vi "Dashboard 2022.vi"() -> ()   [LabVIEW 2020]
uses:
  <vilib>/event_ctls.llb/eventvkey.ctl
  <vilib>/Rock Robotics/WPI/Dashboard/WPI_DashboardLogging Global.vi
  <vilib>/Utility/miscctls.llb/LVRowAndColumnTypeDef.ctl
  <vilib>/Rock Robotics/Network Tables/NT Read Numeric Array.vi
panel:
  in  "Camera Settings Right":T1={"Frame Rate"=30, "Compression"=30, "Size"=1, "DB Camera Config"=FALSE} {"Frame Rate" scale=1.0..30.0; "Compression" scale=100.0..-1.0; "Size" items=["640x480", "320x240", "160x120"]}
  in  "Camera Name Right":string(combo)="No Camera Selection"
  out "Camera Perf":string
  in  "Camera Settings":T1={"Frame Rate"=30, "Compression"=30, "Size"=1, "DB Camera Config"=FALSE} {"Frame Rate" scale=1.0..30.0; "Compression" scale=100.0..-1.0; "Size" items=["640x480", "320x240", "160x120"]}
  in  "TCP":refnum<k5>
  in  "Rec Mode":enum32{"Stop", "Record", "Playback"}(radio)
  out "Robot IP":string
  out "Image Message":string="Timeout in Camera Communications"
  in  "Dashboard Tab":T2(tab)
  in  "Select Auto":string(combo)="Select Autonomous ..."
  out "NT Connection":bool
  out "MotorChart R":cluster{"Numeric":dbl, "Numeric":dbl}(graph)
  out "MotorChart L":cluster{"Numeric":dbl, "Numeric":dbl}(graph)
  out "MotorSliders R":cluster{"MotorSlide1":dbl, "MotorSlide2":dbl} {"MotorSlide2" scale=-1.0..1.0 scale format="%#_2e"; "MotorSlide1" scale=-1.0..1.0 scale format="%#_2e"}
  out "MotorSliders L":cluster{"MotorSlide1":dbl, "MotorSlide2":dbl} {"MotorSlide2" scale=-1.0..1.0 scale format="%#_2e"; "MotorSlide1" scale=-1.0..1.0 scale format="%#_2e"}
  out "Gyro":dbl(knob) scale=0.0..360.0
  out "JS1 Z":dbl(slide) scale=-1.0..1.0 scale format="%#_2e"
  out "JS1 Graph":cluster{"X":dbl, "Y":dbl}[](graph)
  out "JS1 Buttons":T3
  out "JS2 Z":dbl(slide) scale=-1.0..1.0 scale format="%#_2e"
  out "JS2 Graph":cluster{"X":dbl, "Y":dbl}[](graph)
  out "JS2 Buttons":T3
  out "Mode":T4(ring)=enum."Auto Disabled"
  out "Right Camera Perf":cluster{"Bandwidth (Mbps)":dbl, "FPS":dbl}
  out "Camera Image Right":T5(plugin-control)
  in  "DB/String 9":string
  in  "DB/String 8":string
  in  "DB/String 7":string
  in  "DB/String 6":string
  in  "DB/String 5":string
  in  "DB/String 4":string
  in  "DB/String 3":string
  in  "DB/String 2":string
  in  "DB/String 1":string
  in  "DB/String 0":string
  in  "DB/Slider 0":dbl(slide) scale=0.0..5.0
  in  "DB/Slider 1":dbl(slide) scale=0.0..5.0
  in  "DB/Slider 2":dbl(slide) scale=0.0..5.0
  in  "DB/Slider 3":dbl(slide) scale=0.0..5.0
  out "DB/LED 3":bool
  out "DB/LED 2":bool
  out "DB/LED 1":bool
  out "DB/LED 0":bool
  in  "DB/Button 3":bool
  in  "DB/Button 2":bool
  in  "DB/Button 1":bool
  in  "DB/Button 0":bool caption="New Name"
  in  "Test Slider":dbl(slide) scale=0.0..100.0 scale format="%#_3g"
  in  "On/Off":bool caption="Solenoid"
  in  "Test Name":u16(ring) items=["Select the test to run..."]
  in  "Test Tree":string(tree)
  in  "Motor":cluster{"Value":dbl, "Enable":bool} {"Value" scale=-1.0..1.0 scale format="%#_3g"}
  out "Progress":T6 {"Test Progress" scale=0.0..100.0}
  in  "Rev/Fwd":cluster{"Forward":bool, "Reverse":bool}
  in  "Test Ring":u16(ring) items=["Monochrome", "Color"]
  out "Cmd Status":string
  in  "Execute Command":bool
  in  "Command Params":string[][](table)
  in  "Command Selection":i32(listbox)
  in  "CheckList":i32(listbox)
  out "Tree":string(tree)
  out "Right Speed Chart":dbl(graph)
  out "Left Speed Chart":dbl(graph)
  out "Camera Image":T5(plugin-control)
  out "Background":bool
  in  "Camera Name":string(combo)="No Camera Selection"
  # "HW"
  # "HW"
  # "Joysticks"
  # "Drive Motors"
  # "Front"
  # "Right"
  # "Left"
  # "Back"
  # "This tab is a great place for autonomous settings and robot-specific values.\nPlace controls and indicators inside this tab and match name to\nDashboard Variables on robot. You can also delete this comment."
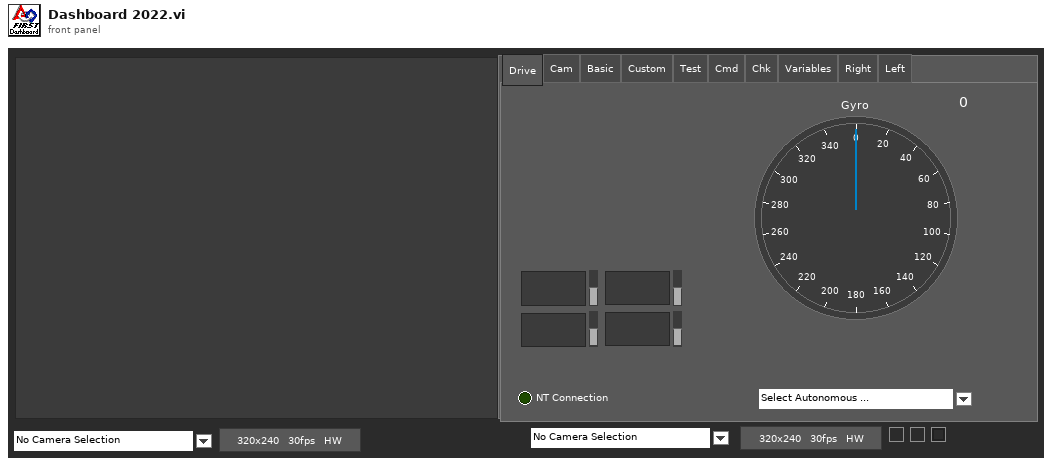
[diagram p1: front panel]
types:
  T1 = cluster{"Frame Rate":i32, "Compression":i32, "Size":u16, "DB Camera Config":bool}
  T2 = enum32{"Drive", "Cam", "Basic", "Custom", "Test", "Cmd", "Chk", "Variables", "Right", "Left"}
  T3 = cluster{bool, bool, bool, bool, bool, bool, bool, bool, bool, bool, bool, bool}
  T4 = enum8{"Tele-Op Disabled", "Tele-Op Enabled", "Auto Disabled", "Auto Enabled", "Test Disabled", "Test Enabled", "Disconnected", "No Code", "E-Stop"}
  T5 = typedef "IMAQ Image.ctl" = refnum<image>
  T6 = cluster{"Test Progress":u8, "Test Progress Text":string}
  T7 = cluster{"Save Path":path, "Interval (s)":dbl, "Keep":i32}
  T8 = enum32{"Drive", "Camera", "Basic", "Custom", "Test", "Commands", "Checklist", "Variables"}
  T9 = typedef "Image Type" = u32
  T10 = cluster{"IDs":cluster{"RPC field ID":u16, "Unique ID":u16}, "String":string}
  T11 = cluster{"Error Strings":string, "Disable Counts":cluster{u16, u16}, "Rail Faults":cluster{u16, u16, u16}, "Robot IP":string, "DB Mode":u8, "Event Info":cluster{"Name":string, "Type":u8, "Number":u16, "Replay":u8}}
  T12 = cluster{"Storage":cluster{"Disk Free":u64, "RAM Block":u32, "RAM free":u32}, "CPU Utilization":cluster{"CPU % ISR":sgl, "CPU % Time Crit":sgl, "CPU % Timed Str":sgl, "CPU % High":sgl, "CPU % Above":sgl, "CPU % Normal":sgl, "CPU % Low":sgl}, "CAN":cluster{"% Bus Utilization":sgl, "Bus Off Cnt":u32, "TX_FIFO Full Cnt":u32, "Receive Error Cnt":u8, "Transmit Error Cnt":u8}, "HID":cluster{"HID Outputs":u32, "Rumble Low":u16, "Rumble High":u16}[]}
  T13 = cluster{"Status bits":cluster{"Test Mode":bool, "Autonomous":bool, "Enabled":bool, "Code Start":bool, "Brownout":bool, "Reserved 2":bool, "Reserved 3":bool, "E-Stop":bool}, "Code Trace":cluster{"Disabled":bool, "TeleOp":bool, "Auto":bool, "Test":bool}, "Controller Type":enum16{"unknown", "cRIO", "roboRio"}, "Code?":enum16{"unknown", "noCode", "code"}, "Battery V":dbl}
  T14 = cluster{"Control Bits":cluster{"TestMode":bool, "Autonomous":bool, "Enabled":bool, "FMS Present":bool, bool, bool, bool, "E-Stop":bool}, "Team Station ":u8, "Countdown":sgl, "Joystick Values":cluster{"Axes":dbl[], "Buttons":bool[], "POVs":i16[]}[]}
  T15 = cluster{"Axes":dbl[], "Buttons":bool[], "POVs":i16[]}[]
  T16 = cluster{"Axes":dbl[], "Buttons":bool[], "POVs":i16[]}
  T17 = cluster{"Buttons[0]":bool, "Buttons[1]":bool, "Buttons[2]":bool, "Buttons[3]":bool, "Buttons[4]":bool, "Buttons[5]":bool, "Buttons[6]":bool, "Buttons[7]":bool, "Buttons[8]":bool, "Buttons[9]":bool, "Buttons[10]":bool, "Buttons[11]":bool}
  T18 = cluster{"Camera Image":refnum<vi>, "Dashboard Tab":refnum<vi>, "Background":refnum<vi>, "Rec Mode":refnum<vi>, "Test Slider":refnum<vi>, "On/Off ":refnum<vi>, "Test Ring":refnum<vi>, "Rev/Fwd":refnum<vi>, "Test Name":refnum<vi>, "Motor":refnum<vi>, "Progress":refnum<vi>, "CheckList":refnum<vi>, "Tree":refnum<vi>, "Test Tree":refnum<vi>, "Command Params":refnum<vi>, "Command Selection":refnum<vi>, "Execute Command":refnum<vi>, "Cmd Status":refnum<vi>, "Camera Settings":refnum<vi>, "Camera Name":refnum<vi>, "Camera Perf":refnum<vi>, "Camera Settings Right":refnum<vi>, "Camera Name Right":refnum<vi>, "Camera Image Right":refnum<vi>}
  T19 = cluster{"Global Rectangle":i32[], "Contours":cluster{"Contour Type":u32, "ROI Type":u32, "Points":i32[]}[]}
  T20 = cluster{"Camera Name":string, string, "Saved DB Images Info":cluster{"Save Path":path, "Interval (s)":dbl, "Keep":i32}}
  T21 = cluster{"Camera Name Right":string, string, "Saved DB Images Info":cluster{"Save Path":path, "Interval (s)":dbl, "Keep":i32}}
  T22 = cluster{"Operation":enum16{"Update", "Clear"}, "Color Box":u32}[]
  T23 = typedef "eventvkey.ctl" = enum16{"ASCII", "Enter", "Return", "Shift", "Ctrl", "Alt", "Cmd", "Opt", "Caps", "NumLock", "Clear", "Break", "Up", "Down", "Left", "Right", "Insert", "Delete", "Home", "End", "PageUp", "PageDown", "Escape", "Help", "Pause", "ScrollLock", "F1", "F2", "F3", "F4", "F5", "F6", "F7", "F8", "F9", "F10", "F11", "F12", "F13", "F14", "F15", "F16", "F17", "F18", "F19", "F20", "F21", "F22", "F23", "F24", "Play", "VolumeUp", "VolumeDown", "Mute", "Two Byte Char"}
  T24 = cluster{"Image Size":bool, "Image Type":bool, "Pixel Value":bool, "ROI Information":bool, "Zoom Factor":bool}
  T25 = cluster{"Operation":enum16{"Update", "Clear"}, "Color Box":u32}
  T26 = typedef "LVRowAndColumnTypeDef.ctl" = cluster{"Row":i32, "Column":i32}
  T27 = cluster{"Shift":bool, "Ctrl":bool, "Alt":bool, "Cmd":bool, "Opt":bool}
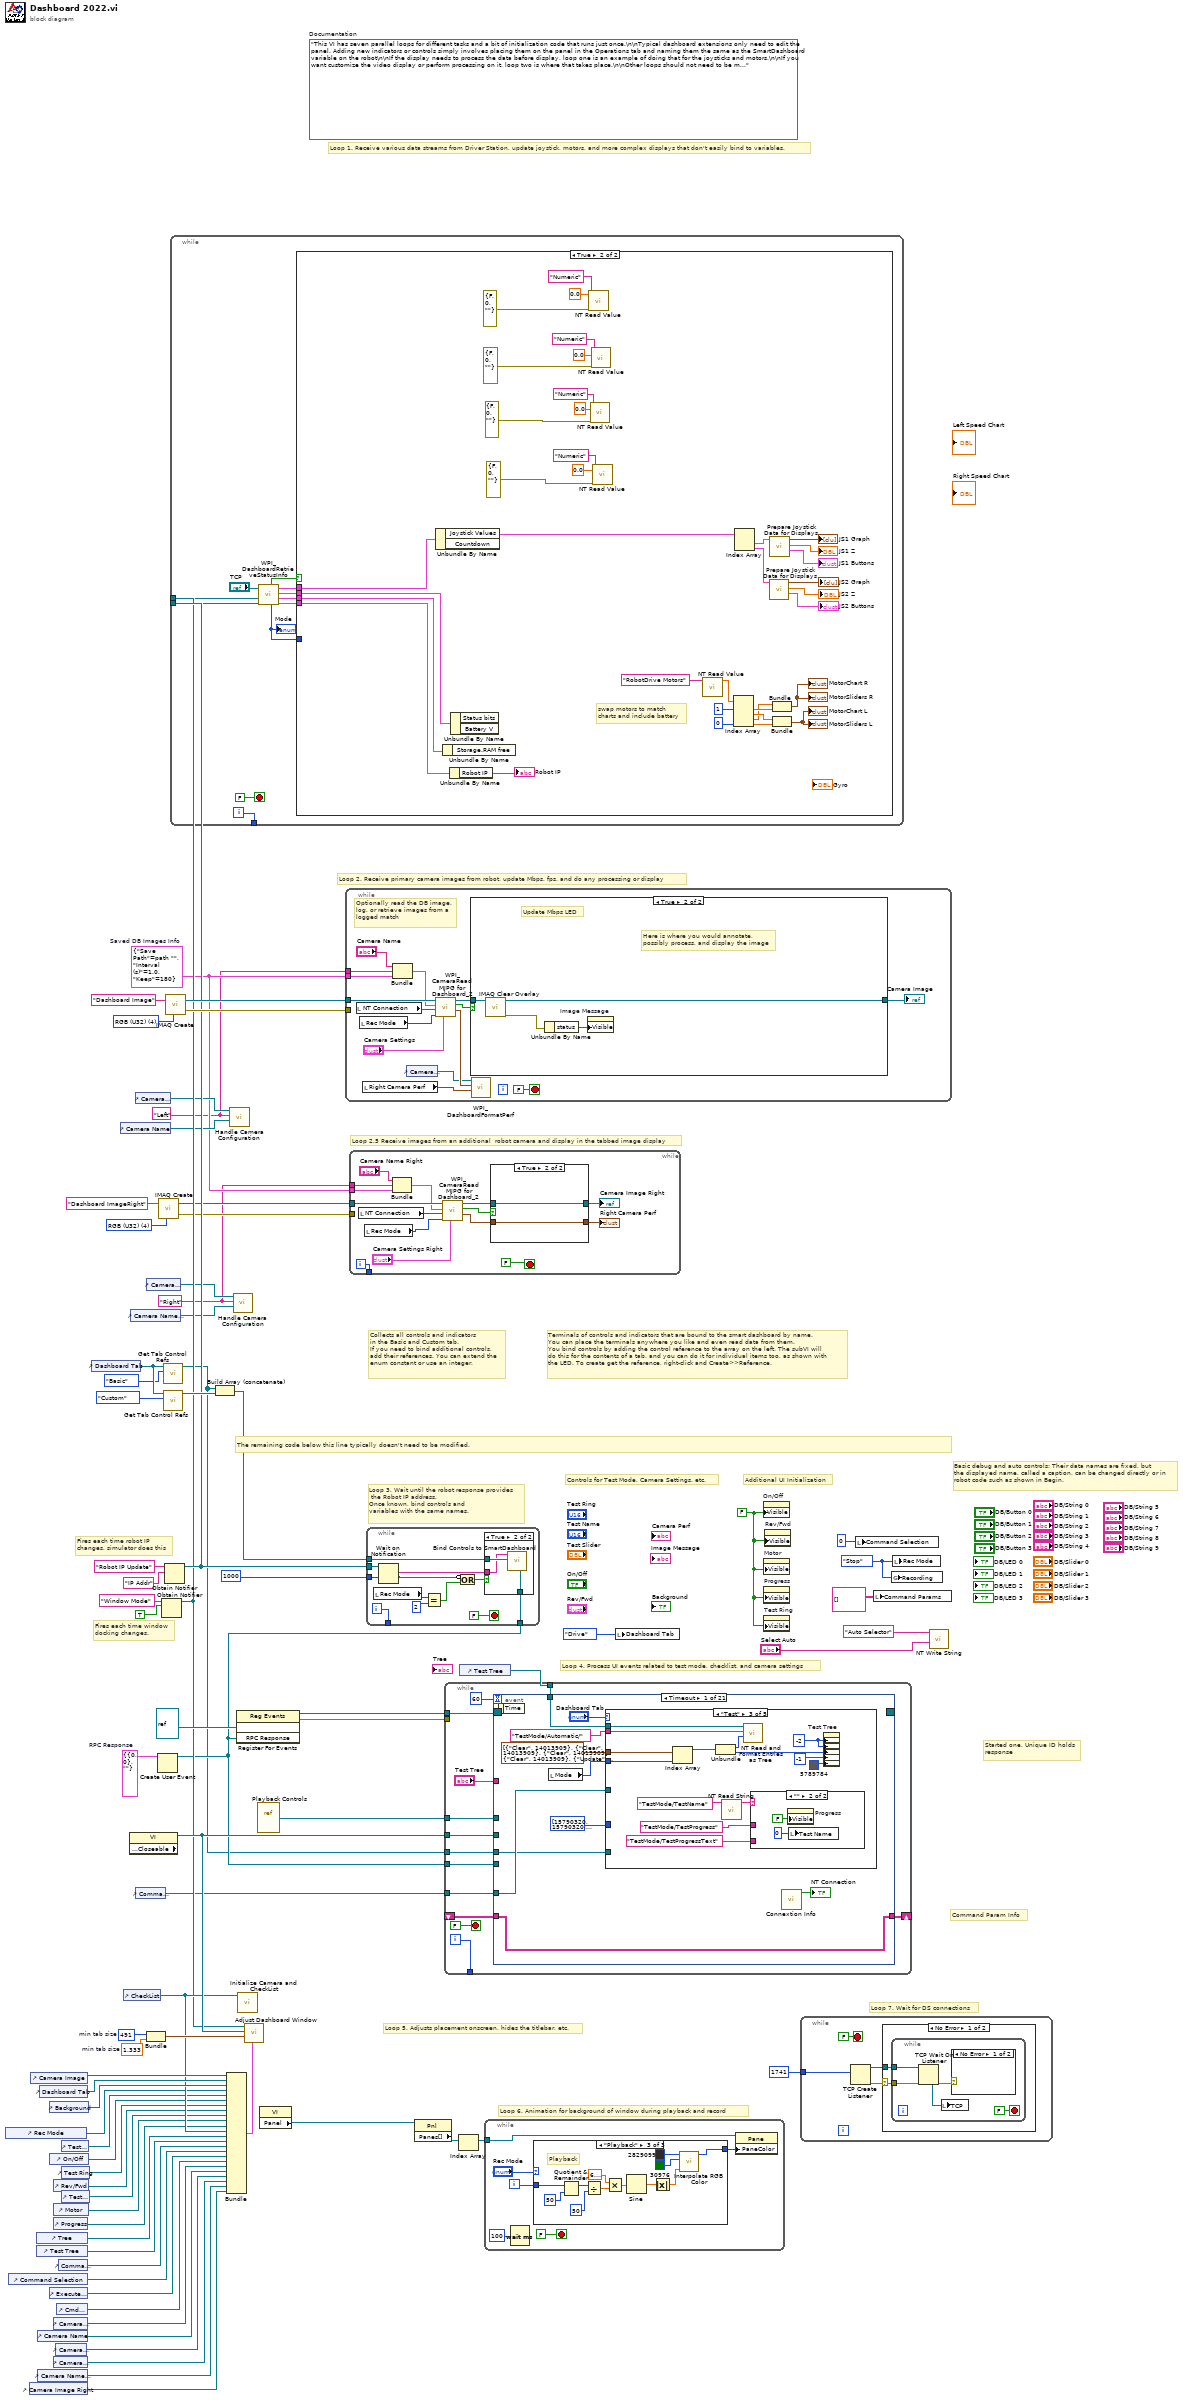
[diagram p0: block diagram]
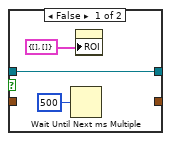
[diagram p2: hidden frame]
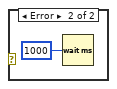
[diagram p3: hidden frame]
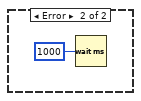
[diagram p4: hidden frame]
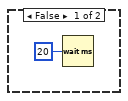
[diagram p5: hidden frame]
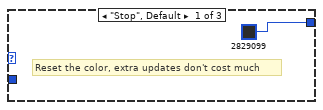
[diagram p6: hidden frame]
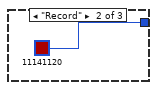
[diagram p7: hidden frame]
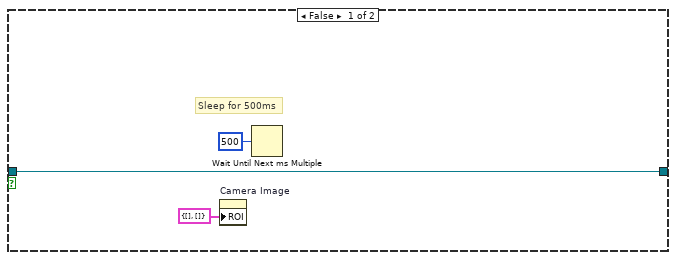
[diagram p9: hidden frame]
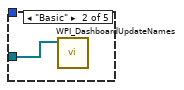
[diagram p11: hidden frame]
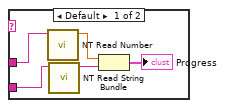
[diagram p12: hidden frame]
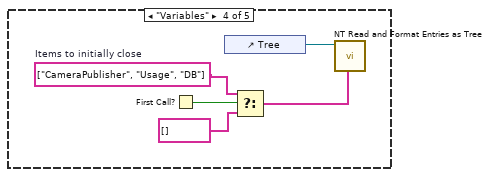
[diagram p13: hidden frame]
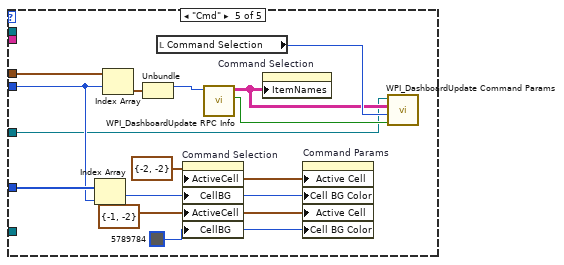
[diagram p14: hidden frame]
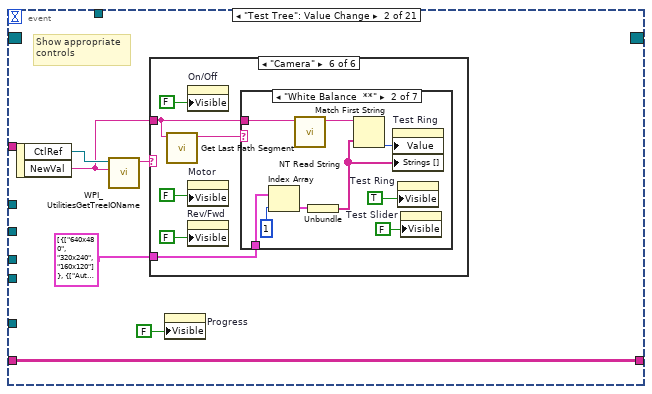
[diagram p15: hidden frame]
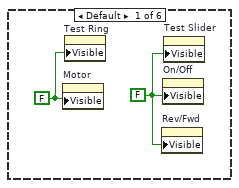
[diagram p16: hidden frame]
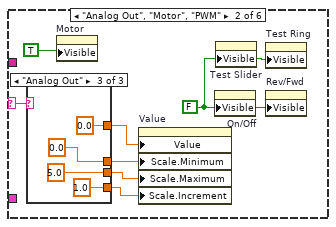
[diagram p17: hidden frame]
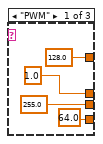
[diagram p18: hidden frame]
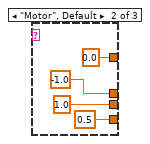
[diagram p19: hidden frame]
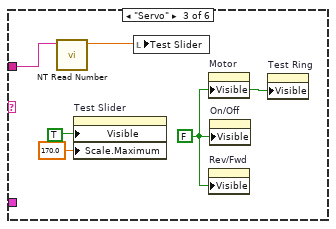
[diagram p20: hidden frame]
diagram:
  w3 = T7 {"Save Path"=path "", "Interval (s)"=1.0, "Keep"=180}  # Saved DB Images Info
  w2 = "Right"
  w1 = "Left"
  w13 = T9 4 items=["Grayscale (U8)", "Grayscale (I16)", "Grayscale (SGL)", "Complex (CSG)", "RGB (U32)", "HSL (U32)", "RGB (U64)"] ("Image Type")
  w29 = T10 {"IDs"={"RPC field ID"=0, "Unique ID"=0}, "String"=""}  # RPC Response
  w52 = 491  # min tab size
  w51 = 1.333  # min tab size
  w59 = enum32{"Stop", "Record", "Playback"}."Stop" ("Rec Mode")
  w36 = FALSE ("Visible")
  (unwired) "This VI has seven parallel loops for different tasks and a bit of initialization code that runs just once.\n\nTypical dashboard extensions only need to edit the panel. Adding new indicators or controls simply involves placing them on the panel in the Operations tab and naming them the same as the SmartDashboard variable on the robot\n\nIf the display needs to process the data before display, loop one is an example of doing that for the joysticks and motors.\n\nIf you want customize the video display or perform processing on it, loop two is where that takes place.\n\nOther loops should not need to be modified. They are pretty standard, and document the task they perform."  # Documentation
  w76 = T9 4 items=["Grayscale (U8)", "Grayscale (I16)", "Grayscale (SGL)", "Complex (CSG)", "RGB (U32)", "HSL (U32)", "RGB (U64)"] ("Image Type")
  # "Loop 2.5 Receive images from an additional  robot camera and display in the tabbed image display"
  # "Command Param Info"
  # "Started one, Unique ID holds\nresponse"
  # "Loop 7. Wait for DS connections"
  # "Basic debug and auto controls: Their data names are fixed, but\nthe displayed name, called a caption, can be changed directly or in\nrobot code such as shown in Begin."
  # "Controls for Test Mode, Camera Settings, etc."
  # "Additional UI Initialization"
  # "Loop 6. Animation for background of window during playback and record"
  # "Fires each time robot IP\nchanges, simulator does this"
  # "Fires each time window\ndocking changes."
  # "Collects all controls and indicators\nin the Basic and Custom tab.\nIf you need to bind additional controls,\nadd their references. You can extend the\nenum constant or use an integer."
  # "The remaining code below this line typically doesn't need to be modified."
  # "Loop 4. Process UI events related to test mode, checklist, and camera settings"
  # "Terminals of controls and indicators that are bound to the smart dashboard by name.\nYou can place the terminals anywhere you like and even read data from them.\nYou bind controls by adding the control reference to the array on the left. The subVI will\ndo this for the contents of a tab, and you can do it for individual items too, as shown with\nthe LED. To create get the reference, right-click and Create>>Reference."
  # "Loop 3. Wait until the robot response provides\n the Robot IP address.\nOnce known, bind controls and\nvariables with the same names."
  # "Loop 5. Adjusts placement onscreen, hides the titlebar, etc."
  # "Loop 1. Receive various data streams from Driver Station, update joystick, motors, and more complex displays that don't easily bind to variables."
  # "Loop 2. Receive primary camera images from robot, update Mbps, fps, and do any processing or display"
  n1 = control-ref of="Rec Mode"() -> (w42:refnum<vi>)
  n2 = control-ref of="Command Selection"() -> (w28:refnum<vi>)
  n3 = control-ref of="Camera Image Right"() -> (w6:refnum<vi>)
  n4 = control-ref of="Camera Image"() -> (w54:refnum<vi>)
  n5 = control-ref of="Tree"() -> (w46:refnum<vi>)
  n6 = control-ref of="Test Tree"() -> (w45:refnum<vi>)
  n7 = control-ref of="Camera Name"() -> (w19:refnum<vi>)
  n8 = control-ref of="Camera Name Right"() -> (w7:refnum<vi>)
  n9 = control-ref of="Dashboard Tab"() -> (w53:refnum<vi>)
  n10 = control-ref of="Execute Command"() -> (w30:refnum<vi>)
  n11 = control-ref of="Background"() -> (w49:refnum<vi>)
  n12 = control-ref of="On/Off"() -> (w40:refnum<vi>)
  n13 = control-ref of="Progress"() -> (w37:refnum<vi>)
  n14 = control-ref of="Camera Settings"() -> (w20:refnum<vi>)
  n15 = control-ref of="Camera Settings Right"() -> (w8:refnum<vi>)
  n16 = control-ref of="Rev/Fwd"() -> (w38:refnum<vi>)
  n17 = control-ref of="Motor"() -> (w43:refnum<vi>)
  n18 = control-ref of="Camera Perf"() -> (w18:refnum<vi>)
  n19 = control-ref of="Cmd Status"() -> (w24:refnum<vi>)
  n20 = control-ref of="Command Params"() -> (w31:refnum<vi>)
  n21 = control-ref of="Test Slider"() -> (w41:refnum<vi>)
  n22 = control-ref of="Test Ring"() -> (w39:refnum<vi>)
  n23 = control-ref of="Test Name"() -> (w44:refnum<vi>)
  n24 = control-ref of="Dashboard Tab"() -> (w57:refnum<vi>)
  n25 = control-ref of="Camera Name"() -> (w21:refnum<vi>)
  n26 = control-ref of="CheckList"() -> (w47:refnum<vi>)
  n27 = property class="VI" props=["Front Panel.Closeable"]() -> (reference out=w58:refnum<vi>)  [unwired: 2 in, 2 out]
  n28 = control-ref of="Camera Name Right"() -> (w9:refnum<vi>)
  n29 = control-ref of="Camera Settings"() -> (w22:refnum<vi>)
  n30 = control-ref of="Command Params"() -> (w23:refnum<vi>)
  n31 = control-ref of="Camera Settings Right"() -> (w10:refnum<vi>)
  n32 = Bundle("min tab size"=w52, "min tab size"=w51) -> (w50:cluster{"min tab size":i32, "min tab size":dbl})  [unwired: 1 in]
  n33 = Create User Event(user event datatype=w29) -> (user event=w25:refnum<user-event>)  [unwired: 1 in, 1 out]
  n34 = call "IMAQ Create"("Image Name"="Dashboard ImageRight", "Image Type"=w13) -> ("New Image"=w12:T5, "error out"=w11:errorcluster)  [unwired: 2 in, 1 out]
  n35 = Obtain Notifier(name (unnamed)="Window Mode", notification data type=TRUE) -> (notifier out=w34:refnum<notifier>)  [unwired: 2 in, 2 out]
  n36 = call <vilib>:"Get Tab Control Refs.vi"("Page Index"=T8."Basic" ("Dashboard Tab"), "TabControl in"=w57) -> ("ControlsOnPage"=w17:refnum<vi>[])  [unwired: 9 in]
  n37 = call <vilib>:"Get Tab Control Refs.vi"("Page Index"=T8."Custom" ("Dashboard Tab"), "TabControl in"=w57) -> ("ControlsOnPage"=w56:refnum<vi>[])  [unwired: 9 in]
  n38 = Obtain Notifier(name (unnamed)="Robot IP Update", notification data type="IP Addr" ("name (unnamed)")) -> (notifier out=w35:refnum<notifier>)  [unwired: 2 in, 2 out]
  n39 = call "IMAQ Create"("Image Name"="Dashboard Image", "Image Type"=w76) -> ("New Image"=w74:T5, "error out"=w73:errorcluster)  [unwired: 2 in, 1 out]
  n40 = while {
    tunnel: [w86] -> _
    tunnel: w35 -> [w80]
    tunnel: w34 -> [w77]
    i -> [w86]
    stop <- FALSE stop-if-true
    n41 = call <vilib>:"WPI_DashboardRetrieveStatusInfo.vi"("Binding Refnum"=w80, "Window Mode Notifier"=w77, "TCP Cnx"="TCP") -> ("Power and Errors"=w81:T11, "Robot Metrics"=w84:T12, "Status Info"=w85:T13, "Control Info"=w82:T14, "Robot Mode"=w79:T4, "Process?"=w83:bool)  [unwired: 3 in]
    "Mode" <- w79
    n42 = case shown="True" w83 {
      tunnel: w85 -> [_ w124]
      tunnel: w84 -> [_ w123]
      tunnel: w82 -> [_ w122]
      tunnel: w81 -> [_ w121]
      tunnel: w79 -> [_ _]
      frame False {
        n43 = Wait (ms)(milliseconds to wait=u32 20) -> ()  [unwired: 1 out]
      }
      frame True {
        # "swap motors to match\ncharts and include battery"
        n44 = Unbundle By Name(w122) -> ("Joystick Values"=w112:T15)  [unwired: 1 out]
        n45 = Unbundle By Name(w123) -> ()  [unwired: 1 out]
        n46 = Unbundle By Name(w121) -> ("Robot IP"=→"Robot IP":string)
        n47 = Unbundle By Name(w124) -> ()  [unwired: 2 out]
        n48 = call-poly <vilib>:"NT Read Value.vi"("error in"=errorcluster {"status"=FALSE, "code"=0, "source"=""}, "Default Value"=0.0, "Name"="Numeric") -> ()  [unwired: 7 in, 2 out]
        n49 = call-poly <vilib>:"NT Read Value.vi"("error in"=errorcluster {"status"=FALSE, "code"=0, "source"=""}, "Default Value"=0.0, "Name"="Numeric") -> ()  [unwired: 7 in, 2 out]
        n50 = call-poly <vilib>:"NT Read Value.vi"("error in"=errorcluster {"status"=FALSE, "code"=0, "source"=""}, "Default Value"=0.0, "Name"="Numeric") -> ()  [unwired: 7 in, 2 out]
        n51 = call-poly <vilib>:"NT Read Value.vi"("error in"=errorcluster {"status"=FALSE, "code"=0, "source"=""}, "Default Value"=0.0, "Name"="Numeric") -> ()  [unwired: 7 in, 2 out]
        n52 = call-poly <vilib>:"NT Read Value.vi"("Name"="RobotDrive Motors") -> ("Numeric Array"=w102:dbl[])  [unwired: 9 in, 1 out]
        n53 = Index Array(array=w102, index #1=1, index #4=0) -> (element #1=w116:dbl, element #2=w117:dbl, element #3=w115:dbl, element #4=w120:dbl)  [unwired: 2 in]
        n54 = Index Array(array=w112) -> (element #1=w111:T16, element #2=w107:T16)  [unwired: 2 in]
        n55 = call "Prepare Joystick Data for Displays.vi"("Joystick Values"=w107) -> ("Buttons"=→"JS2 Buttons":T17, "Z Axis"=→"JS2 Z":dbl, "Cartesian Data"=→"JS2 Graph":cluster{"X axis":dbl, "X axis":dbl}[])  [unwired: 8 in]
        n56 = call "Prepare Joystick Data for Displays.vi"("Joystick Values"=w111) -> ("Buttons"=→"JS1 Buttons":T17, "Z Axis"=→"JS1 Z":dbl, "Cartesian Data"=→"JS1 Graph":cluster{"X axis":dbl, "X axis":dbl}[])  [unwired: 8 in]
        n57 = Bundle("Numeric"=w115, "Numeric"=w116) -> (→"MotorChart R" →"MotorSliders R":cluster{"Numeric":dbl, "Numeric":dbl})  [unwired: 1 in]
        n58 = Bundle("Numeric"=w117, "Numeric"=w120) -> (→"MotorChart L" →"MotorSliders L":cluster{"Numeric":dbl, "Numeric":dbl})  [unwired: 1 in]
      }
    }
  }
  n59 = Build Array (concatenate)(w17, w56) -> (w55:refnum<vi>[])
  n60 = Bundle("Camera Image"=w54, "Dashboard Tab"=w53, "Background"=w49, "Rec Mode"=w42, "Test Slider"=w41, "On/Off"=w40, "Test Ring"=w39, "Rev/Fwd"=w38, "Test Name"=w44, "Motor"=w43, "Progress"=w37, "CheckList"=w47, "Tree"=w46, "Test Tree"=w45, "Command Params"=w31, "Command Selection"=w28, "Execute Command"=w30, "Cmd Status"=w24, "Camera Settings"=w20, "Camera Name"=w19, "Camera Perf"=w18, "Camera Settings Right"=w8, "Camera Name Right"=w7, "Camera Image Right"=w6) -> (w48:T18)  [unwired: 1 in]
  n61 = call "Handle Camera Configuration.vi"("CameraNameRef"=w21, "Display Name"=w1, "ClusterRef"=w22) -> ()  [unwired: 9 in]
  n62 = call "Handle Camera Configuration.vi"("CameraNameRef"=w9, "Display Name"=w2, "ClusterRef"=w10) -> ()  [unwired: 9 in]
  n63 = register-events(refnum<vi> refnum, w25) -> (reference out=w63:refnum<event-registration>, error out=w62:errorcluster)  [unwired: 2 in]
  n64 = call "Initialize Camera and CheckList.vi"("ListBox in"=w47) -> ()  [unwired: 11 in]
  n65 = call "Adjust Dashboard Window.vi"("Sizing Refnums"=w48, "Size Constraints"=w50, "VI"=w58, "WIn Mode"=w34) -> ()  [unwired: 8 in]
  n66 = vi-ref "Playback Controls.vi"() -> (w64:refnum<vi>)
  n67 = property class="VI"() -> ("Panel"=w66:refnum<vi>)  [unwired: 2 in, 2 out]
  n68 = while {
    tunnel: w74 -> [w138]
    tunnel: w73 -> [_]
    tunnel: w3 -> [w131]
    tunnel: w1 -> [w128]
    stop <- FALSE stop-if-true
    # "Optionally read the DB image,\nlog, or retrieve images from a\nlogged match"
    n69 = local read "NT Connection"() -> (w132:bool)
    n70 = local read "Rec Mode"() -> (w135:enum32{"Stop", "Record", "Playback"})
    n71 = local read "Right Camera Perf"() -> (w126:cluster{"Bandwidth (Mbps)":dbl, "FPS":dbl})
    n72 = Bundle("Camera Name"="Camera Name", w128, "Saved DB Images Info"=w131) -> (w130:T20)  [unwired: 1 in]
    n73 = control-ref of="Camera Perf"() -> (w125:refnum<vi>)
    n74 = call <vilib>:"WPI_CameraRead MJPG for Dashboard_2.vi"("Camera Settings"="Camera Settings", "Rec Mode"=w135, "NT Connection"=w132, "Capture Info"=w130, "Image in"=w138) -> ("perf info"=w127:cluster{"Bandwidth (Mbps)":dbl, "fps":dbl}, "Active"=w136:bool, "Image\\ out"=w137:T5)  [unwired: 4 in]
    n75 = case shown="True" w136 {
      tunnel: w137 -> [w141 w144]
      tunnel: [w141 w143] -> w133
      frame False {
        # "Sleep for 500ms"
        n76 = property on="Camera Image" class="ImageControl"("ROI"=T19 {"Global Rectangle"=[], "Contours"=[]}) -> ()  [unwired: 2 in, 2 out]
        n77 = Wait Until Next ms Multiple(millisecond multiple=u32 500) -> ()  [unwired: 1 out]
      }
      frame True {
        # "Here is where you would annotate,\npossibly process, and display the image"
        # "Update Mbps LED"
        n78 = call "IMAQ Clear Overlay"("Image"=w144) -> ("error out"=w145:errorcluster, "Image Out"=w143:T5)  [unwired: 2 in, 7 out]
        n79 = Unbundle By Name(w145) -> ("status"=w146:bool)
        n80 = property on="Image Message" class="Str"("Visible"=w146) -> ()  [unwired: 2 in, 2 out]
      }
    }
    "Camera Image" <- w133
    n81 = call <vilib>:"WPI_DashboardFormatPerf.vi"("Right Camera Perf"=w126, "Performance"=w127, "String in"=w125) -> ()  [unwired: 9 in]
  }
  n82 = while {
    tunnel: w12 -> [w161]
    tunnel: w11 -> [_]
    tunnel: [w156] -> _
    tunnel: w3 -> [w152]
    tunnel: w2 -> [w149]
    i -> [w156]
    stop <- FALSE stop-if-true
    n83 = local read "NT Connection"() -> (w153:bool)
    n84 = local read "Rec Mode"() -> (w160:enum32{"Stop", "Record", "Playback"})
    n85 = Bundle("Camera Name Right"="Camera Name Right", w149, "Saved DB Images Info"=w152) -> (w151:T21)  [unwired: 1 in]
    n86 = call <vilib>:"WPI_CameraRead MJPG for Dashboard_2.vi"("Camera Settings"="Camera Settings Right", "Rec Mode"=w160, "NT Connection"=w153, "Capture Info"=w151, "Image in"=w161) -> ("perf info"=w147:cluster{"Bandwidth (Mbps)":dbl, "fps":dbl}, "Active"=w155:bool, "Image\\ out"=w158:T5)  [unwired: 4 in]
    n87 = case shown="True" w155 {
      tunnel: w158 -> [w163 w166]
      tunnel: [w163 w166] -> w154
      tunnel: [_ w165] -> w148
      tunnel: w147 -> [_ w165]
      frame False {
        n88 = Wait Until Next ms Multiple(millisecond multiple=u32 500) -> ()  [unwired: 1 out]
        n89 = property on="Camera Image Right" class="ImageControl"("ROI"=T19 {"Global Rectangle"=[], "Contours"=[]}) -> ()  [unwired: 2 in, 2 out]
      }
      frame True {
      }
    }
    "Camera Image Right" <- w154
    "Right Camera Perf" <- w148
  }
  n90 = while {
    tunnel: w55 -> [w178]
    tunnel: w35 -> [w176]
    tunnel: [w174] -> _
    tunnel: u32 1000 ("milliseconds to wait") -> [w173]
    tunnel: w25 -> [w167]
    i -> [w174]
    stop <- FALSE stop-if-true
    n91 = local read "Rec Mode"() -> (w169:enum32{"Stop", "Record", "Playback"})
    n92 = Wait on Notification(notifier=w176, timeout in ms (-1)=w173) -> (notification=w175:string, timed out?=w171:bool)  [unwired: 2 in, 2 out]
    n93 = Equal?(x=w169, y=u16 2 ("Rec Mode")) -> (x = y?=w170:bool)
    n94 = Compound Arithmetic op=OR(invert w171, w170) -> (w172:bool)
    n95 = case shown="True" w172 {
      tunnel: w178 -> [_ w181]
      tunnel: w175 -> [_ w180]
      tunnel: w167 -> [_ w179]
      frame False {
      }
      frame True {
        n96 = call <vilib>:"Bind Controls to SmartDashboard.vi"("RPC ref"=w179, "Bound Control Refs"=w181, "Server IP Address"=w180) -> ()  [unwired: 9 in]
      }
    }
  }
  n97 = property class="Pnl"(reference=w66) -> ("Panes[]"=w67:refnum<vi>[])  [unwired: 1 in, 2 out]
  n98 = Index Array(array=w67) -> (element=w65:refnum<vi>)  [unwired: 1 in]
  n99 = control-ref of="Test Tree"() -> (w68:refnum<vi>)
  n100 = while {
    tunnel: [w191] -> _
    tunnel: w68 -> [w190]
    tunnel: w64 -> [w189]
    tunnel: w63 -> [w188]
    tunnel: w62 -> [_]
    tunnel: w58 -> [w187]
    tunnel: w25 -> [w186]
    tunnel: w23 -> [w185]
    shift-right: [w184] -> _
    shift-left: _ -> [w183]
    tunnel: w17 -> [w182]
    i -> [w191]
    stop <- FALSE stop-if-true
    n101 = event shown="[0] Timeout" {
      selector: w188 -> [_ _ _ _ _ _ _ _ _ _ _ _ _ _ _ _ _ _ _ _ _]
      dyn-events: [_ _ _ _ _ _ _ _ _ _ _ _ _ _ _ _ w451 _ _ _ _] -> _
      timeout: u32 60 ("milliseconds to wait") -> [_ _ _ _ _ _ _ _ _ _ _ _ _ _ _ _ _ _ _ _ _]
      tunnel: w190 -> [w203 _ _ _ _ _ _ _ _ _ _ _ _ _ _ _ _ _ _ _ _]
      tunnel: "Test Tree" -> [_ _ _ _ _ _ _ _ _ _ _ w418 w426 w428 w432 w440 _ _ _ _ _]
      tunnel: w189 -> [_ _ _ _ _ _ _ _ _ _ _ _ _ _ _ _ w453 _ w471 _ _]
      tunnel: w187 -> [_ _ _ _ _ _ _ _ _ _ _ _ _ _ _ _ w449 _ _ _ _]
      tunnel: w186 -> [_ _ _ _ _ _ _ _ _ _ _ _ _ _ _ _ w447 _ _ _ _]
      tunnel: w185 -> [w198 _ _ _ _ _ w369 _ _ _ _ _ _ _ _ _ _ _ _ _ _]
      tunnel: [w197 w246 w348 w353 w362 w366 w367 w376 w386 w393 w405 w417 w424 w427 w431 w439 w446 w466 w468 w472 w485] -> w184
      tunnel: w183 -> [w197 w246 w348 w353 w362 w366 w367 _ _ w393 w405 w417 w424 w427 w431 w439 w446 w466 w468 w472 w485]
      tunnel: w182 -> [w195 _ _ _ _ _ _ _ _ _ _ _ _ _ _ _ _ _ _ _ _]
      event Timeout {
        n102 = event-data() -> ()  [unwired: 1 in, 1 out]
        n103 = local read "Mode"() -> (w200:T4)
        n104 = case shown="\"Test\"" "Dashboard Tab" {
          tunnel: w203 -> [_ _ w219 _ _]
          tunnel: "TestMode/Automatic/" ("Name Pattern") -> [_ _ w218 _ _]
          tunnel: T22 [{"Operation"=enum."Clear", "Color Box"=14013909}, {"Operation"=enum."Clear", "Color Box"=14013909}, {"Operation"=enum."Clear", "Color Box"=14013909}, {"Operation"=enum."Clear", "Color Box"=14013909}, {"Operation"=enum."Update", "Color Box"=14013909}, {"Operation"=enum."Update", "Color Box"=16777215}, {"Operation"=enum."Clear", "Color Box"=14013909}, {"Operation"=enum."Clear", "Color Box"=14013909}, {"Operation"=enum."Clear", "Color Box"=14013909}] -> [_ _ w211 _ w239]
          tunnel: w200 -> [_ _ w210 _ w238]
          tunnel: u32[] [15790320, 15790320, 15790320, 15790320, 16777215, 16777215, 15790320, 15790320, 15790320] -> [_ _ _ _ w244]
          tunnel: w198 -> [_ _ _ _ w232]
          tunnel: w195 -> [_ w205 _ _ _]
          frame "Custom", Default {
          }
          frame "Basic" {
            n105 = call <vilib>:"WPI_DashboardUpdateNames.vi"("Controls on Tab"=w205) -> ()  [unwired: 11 in]
          }
          frame "Test" {
            w217 = -2 ("Active Item:Row Number")
            n106 = Index Array(array=w211, index=w210) -> (element=w212:T25)
            n107 = Unbundle(w212) -> ("Operation"=w213:enum16{"Update", "Clear"}, "Color Box"=w214:u32)
            n108 = call <vilib>:"NT Read String.vi"("Name"="TestMode/TestName") -> ("String"=w208:string)  [unwired: 9 in, 1 out]
            n109 = call <vilib>:"NT Read and Format Entries as Tree.vi"("Operation"=w213, "Name Pattern"=w218, "Tree Refnum"=w219) -> ()  [unwired: 7 in, 2 out]
            n110 = case shown="\"\"" w208 {
              tunnel: "TestMode/TestProgress" ("Name") -> [w221 _]
              tunnel: "TestMode/TestProgressText" ("Name") -> [w220 _]
              frame Default {
                n111 = call <vilib>:"NT Read Number.vi"("Name"=w221) -> ("Numeric"=w222:dbl)  [unwired: 9 in, 1 out]
                n112 = call <vilib>:"NT Read String.vi"("Name"=w220) -> ("String"=w223:string)  [unwired: 9 in, 1 out]
                n113 = Bundle("Numeric"=w222, "String"=w223) -> (→"Progress":cluster{"Numeric":dbl, "String":string})  [unwired: 1 in]
              }
              frame "" {
                n114 = property on="Progress" class="Clust (strict)"("Visible"=FALSE) -> ()  [unwired: 2 in, 2 out]
                n115 = local write "Test Name"(u16 0) -> ()
              }
            }
            n116 = property on="Test Tree" class="Tree (strict)"("Active Item Row Number"=w217, "ActiveColNum"=w217, "CellBG"=w214, "Active Item Row Number"=-1 ("Active Item:Row Number"), "CellBG"=u32 5789784 ("Color Box")) -> ()  [unwired: 2 in, 2 out]
          }
          frame "Variables" {
            w229 = string[] ["CameraPublisher", "Usage", "DB"]  # Items to initially close
            n117 = First Call?() -> (First Call?: T/F=w230:bool)
            n118 = control-ref of="Tree"() -> (w231:refnum<vi>)
            n119 = Select(t=w229, s=w230, f=string[] []) -> (s? t:f=w227:string[])
            n120 = call <vilib>:"NT Read and Format Entries as Tree.vi"("Tags to  Close"=w227, "Tree Refnum"=w231) -> ()  [unwired: 8 in, 2 out]
          }
          frame "Cmd" {
            w240 = u32 5789784 ("Color Box")
            w241 = T26 {"Row"=-1, "Column"=-2} ("Active Cell:Active Cell")
            w243 = T26 {"Row"=-2, "Column"=-2} ("Active Cell:Active Cell")
            n121 = Index Array(array=w244, index=w238) -> (element=w242:u32)
            n122 = Index Array(array=w239, index=w238) -> (element=w237:T25)
            n123 = Unbundle(w237) -> ("Operation"=w236:enum16{"Update", "Clear"})  [unwired: 1 out]
            n124 = local read "Command Selection"() -> (w235:i32)
            n125 = property on="Command Selection" class="MCListbox (strict)"("ActiveCell"=w243, "CellBG"=w242, "ActiveCell"=w241, "CellBG"=w240) -> ()  [unwired: 2 in, 2 out]
            n126 = call <vilib>:"WPI_DashboardUpdate RPC Info.vi"("Operation"=w236) -> ("update"=w234:bool, "commands"=w233:string[][])  [unwired: 9 in]
            n127 = property on="Command Selection" class="MCListbox (strict)"("ItemNames"=w233) -> ()  [unwired: 2 in, 2 out]
            n128 = property on="Command Params" class="Tbl (strict)"("Active Cell"=w243, "Cell BG Color"=w242, "Active Cell"=w241, "Cell BG Color"=w240) -> ()  [unwired: 2 in, 2 out]
            n129 = call <vilib>:"WPI_DashboardUpdate Command Params.vi"("Update"=w234, "NewVal"=w235, "Commands"=w233, "Param Tbl"=w232) -> ()  [unwired: 7 in, 1 out]
          }
        }
        n130 = call <vilib>:"Connextion Info.vi"() -> ("Connected"=→"NT Connection":bool)  [unwired: 10 in, 1 out]
      }
      event "Test Tree": Value Change {
        # "Show appropriate\ncontrols"
        n131 = event-data() -> ("CtlRef"=w249:refnum<vi>, "NewVal"=w247:string)  [unwired: 1 in]
        n132 = call <vilib>:"WPI_UtilitiesGetTreeIOName.vi"("NewVal"=w247, "TreeControl in"=w249) -> ("I/O Name"=w250:string)  [unwired: 9 in]
        n133 = case shown="\"Camera\"" w250 {
          selector: w250 -> [_ w257 _ w279 w288 _]
          tunnel: w247 -> [_ _ w276 w278 _ w295]
          tunnel: cluster{string[]}[] [{["640x480", "320x240", "160x120"]}, {["Auto", "Fixed indoor", "Fixed outdoor 1", "Fixed outdoor 2", "Fixed fluorescent 1", "Fixed fluorescent 2", "Hold current"]}, {["Auto", "Flicker-free 50 Hz", "Flicker-free 60 Hz", "Hold current"]}, {["None", "Prioritize frame rate", "Prioritize image quality"]}, {["Monochrome", "Color"]}] -> [_ _ _ _ _ w294]
          frame Default {
            w252 = FALSE ("Visible")
            w251 = FALSE ("Visible")
            n134 = property on="Motor" class="Clust (strict)"("Visible"=w251) -> ()  [unwired: 2 in, 2 out]
            n135 = property on="Test Ring" class="Ring (strict)"("Visible"=w251) -> ()  [unwired: 2 in, 2 out]
            n136 = property on="Rev/Fwd" class="Clust (strict)"("Visible"=w252) -> ()  [unwired: 2 in, 2 out]
            n137 = property on="On/Off" class="Bool (strict)"("Visible"=w252) -> ()  [unwired: 2 in, 2 out]
            n138 = property on="Test Slider" class="Slide (strict)"("Visible"=w252) -> ()  [unwired: 2 in, 2 out]
          }
          frame "Analog Out", "Motor", "PWM" {
            w258 = FALSE ("Visible")
            n139 = case shown="\"Analog Out\"" w257 {
              tunnel: [1.0 ("Value") -1.0 ("Value") 0.0 ("Value")] -> w256
              tunnel: [255.0 ("Value") 1.0 ("Value") 5.0 ("Value")] -> w255
              tunnel: [128.0 ("Value") 0.0 ("Value") 0.0 ("Value")] -> w254
              tunnel: [64.0 ("Value") 0.5 ("Value") 1.0 ("Value")] -> w253
              frame "PWM" {
              }
              frame "Motor", Default {
              }
              frame "Analog Out" {
              }
            }
            n140 = property on="Motor" class="Clust (strict)"("Visible"=TRUE) -> ()  [unwired: 2 in, 2 out]
            n141 = property on="Value" class="Slide (strict)"("Value"=w254, "Scale.Minimum"=w256, "Scale.Maximum"=w255, "Scale.Increment"=w253) -> ()  [unwired: 2 in, 2 out]
            n142 = property on="On/Off" class="Bool (strict)"("Visible"=w258) -> ()  [unwired: 2 in, 2 out]
            n143 = property on="Test Slider" class="Slide (strict)"("Visible"=w258) -> ()  [unwired: 2 in, 2 out]
            n144 = property on="Test Ring" class="Ring (strict)"("Visible"=w258) -> ()  [unwired: 2 in, 2 out]
            n145 = property on="Rev/Fwd" class="Clust (strict)"("Visible"=w258) -> ()  [unwired: 2 in, 2 out]
          }
          frame "Servo" {
            w274 = FALSE ("Visible")
            n146 = call <vilib>:"NT Read Number.vi"("Name"=w276) -> ("Numeric"=w275:dbl)  [unwired: 9 in, 1 out]
            n147 = property on="Test Slider" class="Slide (strict)"("Visible"=TRUE, "Scale.Maximum"=170.0 ("Scale.Range:Maximum")) -> ()  [unwired: 2 in, 2 out]
            n148 = local write "Test Slider"(w275) -> ()
            n149 = property on="Motor" class="Clust (strict)"("Visible"=w274) -> ()  [unwired: 2 in, 2 out]
            n150 = property on="Rev/Fwd" class="Clust (strict)"("Visible"=w274) -> ()  [unwired: 2 in, 2 out]
            n151 = property on="On/Off" class="Bool (strict)"("Visible"=w274) -> ()  [unwired: 2 in, 2 out]
            n152 = property on="Test Ring" class="Ring (strict)"("Visible"=w274) -> ()  [unwired: 2 in, 2 out]
          }
          frame "Relay", "Solenoid" {
            w277 = FALSE ("Visible")
            n153 = property on="Motor" class="Clust (strict)"("Visible"=w277) -> ()  [unwired: 2 in, 2 out]
            n154 = property on="Test Slider" class="Slide (strict)"("Visible"=w277) -> ()  [unwired: 2 in, 2 out]
            n155 = Search and Replace String(input string=w278, search string="/Value  **", replace string="/Direction") -> (result string=w284:string)  [unwired: 5 in, 3 out]
            n156 = property on="Test Ring" class="Ring (strict)"("Visible"=w277) -> ()  [unwired: 2 in, 2 out]
            n157 = call <vilib>:"NT Read String.vi"("Name"=w284) -> ("String"=w282:string)  [unwired: 9 in, 1 out]
            n158 = Equal?(x="Both directions", y=w282) -> (x = y?=w280:bool)
            n159 = Not(x=w280) -> (.not. x?=w281:bool)
            n160 = property on="Rev/Fwd" class="Clust (strict)"("Visible"=w280) -> ()  [unwired: 2 in, 2 out]
            n161 = property on="On/Off" class="Bool (strict)"("Visible"=w281, "Caption.Text"=w279) -> ()  [unwired: 2 in, 2 out]
          }
          frame "Compressor", "Digital Out" {
            w287 = FALSE ("Visible")
            # "Get direction and finish"
            n162 = property on="Motor" class="Clust (strict)"("Visible"=w287) -> ()  [unwired: 2 in, 2 out]
            n163 = property on="Test Slider" class="Slide (strict)"("Visible"=w287) -> ()  [unwired: 2 in, 2 out]
            n164 = property on="Test Ring" class="Ring (strict)"("Visible"=w287) -> ()  [unwired: 2 in, 2 out]
            n165 = property on="On/Off" class="Bool (strict)"("Visible"=TRUE, "Caption.Text"=w288) -> ()  [unwired: 2 in, 2 out]
            n166 = property on="Rev/Fwd" class="Clust (strict)"("Visible"=FALSE) -> ()  [unwired: 2 in, 2 out]
          }
          frame "Camera" {
            n167 = call <vilib>:"Get Last Path Segment.vi"("String in"=w295) -> ("String out"=w296:string)  [unwired: 10 in]
            n168 = property on="On/Off" class="Bool (strict)"("Visible"=FALSE) -> ()  [unwired: 2 in, 2 out]
            n169 = property on="Motor" class="Clust (strict)"("Visible"=FALSE) -> ()  [unwired: 2 in, 2 out]
            n170 = property on="Rev/Fwd" class="Clust (strict)"("Visible"=FALSE) -> ()  [unwired: 2 in, 2 out]
            n171 = case shown="\"White Balance  **\"" w296 {
              tunnel: w295 -> [w302 w311 w320 w329 w338 _ w344]
              tunnel: w294 -> [w300 w308 w317 w326 w335 _ _]
              frame "Size  **" {
                n172 = Index Array(array=w300) -> (element=w299:cluster{string[]})  [unwired: 1 in]
                n173 = call <vilib>:"NT Read String.vi"("Name"=w302) -> ("String"=w301:string)  [unwired: 9 in, 1 out]
                n174 = Unbundle(w299) -> (w297:string[])
                n175 = Match First String(2:w297, 3:w301) -> (0:w298:i32)  [unwired: 1 out]
                n176 = property on="Test Ring" class="Ring (strict)"("Value"=w298, "Strings []"=w297) -> ()  [unwired: 2 in, 2 out]
                n177 = property on="Test Ring" class="Ring (strict)"("Visible"=TRUE) -> ()  [unwired: 2 in, 2 out]
                n178 = property on="Test Slider" class="Slide (strict)"("Visible"=FALSE) -> ()  [unwired: 2 in, 2 out]
              }
              frame "White Balance  **" {
                n179 = Index Array(array=w308, index=1) -> (element=w309:cluster{string[]})
                n180 = call <vilib>:"NT Read String.vi"("Name"=w311) -> ("String"=w310:string)  [unwired: 9 in, 1 out]
                n181 = Unbundle(w309) -> (w306:string[])
                n182 = Match First String(2:w306, 3:w310) -> (0:w305:i32)  [unwired: 1 out]
                n183 = property on="Test Ring" class="Ring (strict)"("Value"=w305, "Strings []"=w306) -> ()  [unwired: 2 in, 2 out]
                n184 = property on="Test Ring" class="Ring (strict)"("Visible"=TRUE) -> ()  [unwired: 2 in, 2 out]
                n185 = property on="Test Slider" class="Slide (strict)"("Visible"=FALSE) -> ()  [unwired: 2 in, 2 out]
              }
              frame "Exposure  **" {
                n186 = Index Array(array=w317, index=2) -> (element=w318:cluster{string[]})
                n187 = call <vilib>:"NT Read String.vi"("Name"=w320) -> ("String"=w319:string)  [unwired: 9 in, 1 out]
                n188 = Unbundle(w318) -> (w314:string[])
                n189 = Match First String(2:w314, 3:w319) -> (0:w315:i32)  [unwired: 1 out]
                n190 = property on="Test Ring" class="Ring (strict)"("Value"=w315, "Strings []"=w314) -> ()  [unwired: 2 in, 2 out]
                n191 = property on="Test Ring" class="Ring (strict)"("Visible"=TRUE) -> ()  [unwired: 2 in, 2 out]
                n192 = property on="Test Slider" class="Slide (strict)"("Visible"=FALSE) -> ()  [unwired: 2 in, 2 out]
              }
              frame "Exposure Priority  **" {
                n193 = Index Array(array=w326, index=3) -> (element=w327:cluster{string[]})
                n194 = call <vilib>:"NT Read String.vi"("Name"=w329) -> ("String"=w328:string)  [unwired: 9 in, 1 out]
                n195 = Unbundle(w327) -> (w323:string[])
                n196 = Match First String(2:w323, 3:w328) -> (0:w324:i32)  [unwired: 1 out]
                n197 = property on="Test Ring" class="Ring (strict)"("Value"=w324, "Strings []"=w323) -> ()  [unwired: 2 in, 2 out]
                n198 = property on="Test Ring" class="Ring (strict)"("Visible"=TRUE) -> ()  [unwired: 2 in, 2 out]
                n199 = property on="Test Slider" class="Slide (strict)"("Visible"=FALSE) -> ()  [unwired: 2 in, 2 out]
              }
              frame "Color Enable  **" {
                n200 = Index Array(array=w335, index=4) -> (element=w336:cluster{string[]})
                n201 = call <vilib>:"NT Read String.vi"("Name"=w338) -> ("String"=w337:string)  [unwired: 9 in, 1 out]
                n202 = Unbundle(w336) -> (w332:string[])
                n203 = Match First String(2:w332, 3:w337) -> (0:w333:i32)  [unwired: 1 out]
                n204 = property on="Test Ring" class="Ring (strict)"("Value"=w333, "Strings []"=w332) -> ()  [unwired: 2 in, 2 out]
                n205 = property on="Test Ring" class="Ring (strict)"("Visible"=TRUE) -> ()  [unwired: 2 in, 2 out]
                n206 = property on="Test Slider" class="Slide (strict)"("Visible"=FALSE) -> ()  [unwired: 2 in, 2 out]
              }
              frame Default {
                n207 = property on="Test Ring" class="Ring (strict)"("Visible"=FALSE) -> ()  [unwired: 2 in, 2 out]
                n208 = property on="Test Slider" class="Slide (strict)"("Visible"=FALSE) -> ()  [unwired: 2 in, 2 out]
              }
              frame "Brightness  **", "Color Level  **", "Compression  **", "FPS  **", "Sharpness  **" {
                n209 = call <vilib>:"NT Read Number.vi"("Name"=w344) -> ("Numeric"=w343:dbl)  [unwired: 9 in, 1 out]
                n210 = local write "Test Slider"(w343) -> ()
                n211 = property on="Test Slider" class="Slide (strict)"("Visible"=TRUE, "Scale.Maximum"=100.0 ("Scale.Range:Maximum")) -> ()  [unwired: 2 in, 2 out]
                n212 = property on="Test Ring" class="Ring (strict)"("Visible"=FALSE) -> ()  [unwired: 2 in, 2 out]
              }
            }
          }
        }
        n213 = property on="Progress" class="Clust (strict)"("Visible"=FALSE) -> ()  [unwired: 2 in, 2 out]
      }
      event "Test Name": Mouse Enter {
        # "Populate the ring with the list of tests"
        n214 = event-data() -> ()  [unwired: 1 in, 1 out]
        n215 = call <vilib>:"NT Read String Array.vi"("Name"="TestMode/TestList") -> ("String Array"=w352:string[])  [unwired: 9 in, 1 out]
        n216 = Build Array (concatenate)("Select the test to run...", w352) -> (w351:string[])
        n217 = property on="Test Name" class="Ring (strict)"("Strings []"=w351) -> ()  [unwired: 2 in, 2 out]
      }
      event "Test Name": Value Change {
        w354 = FALSE ("Visible")
        # "Tell the robot the test name to run"
        n218 = event-data() -> ("NewVal"=w358:u16)  [unwired: 1 in]
        n219 = property on="Test Name" class="Ring (strict)"() -> ("Strings []"=w359:string[])  [unwired: 2 in, 2 out]
        n220 = local write "Progress"(T6 {"Test Progress"=0, "Test Progress Text"=""} ("Progress")) -> ()
        n221 = Index Array(array=w359, index=w358) -> (element=w357:string)
        n222 = call <vilib>:"NT Write String.vi"("String"=w357, "Name"="TestMode/TestName") -> ()  [unwired: 9 in, 1 out]
        n223 = property on="Progress" class="Clust (strict)"("Visible"=TRUE) -> ()  [unwired: 2 in, 2 out]
        n224 = property on="Motor" class="Clust (strict)"("Visible"=w354) -> ()  [unwired: 2 in, 2 out]
        n225 = property on="Test Slider" class="Slide (strict)"("Visible"=w354) -> ()  [unwired: 2 in, 2 out]
        n226 = property on="On/Off" class="Bool (strict)"("Visible"=w354) -> ()  [unwired: 2 in, 2 out]
        n227 = property on="Rev/Fwd" class="Clust (strict)"("Visible"=w354) -> ()  [unwired: 2 in, 2 out]
        n228 = property on="Test Ring" class="Ring (strict)"("Visible"=w354) -> ()  [unwired: 2 in, 2 out]
      }
      event "Select Auto": Mouse Enter {
        # "Populate the combo box with the list of autonomous options"
        n229 = event-data() -> ()  [unwired: 1 in, 1 out]
        n230 = call <vilib>:"NT Read String Array.vi"("Name"="Auto List") -> ("String Array"=w361:string[])  [unwired: 9 in, 1 out]
        n231 = property on="Select Auto" class="CmbBox"("Strings[]"=w361) -> ()  [unwired: 2 in, 2 out]
      }
      event "Select Auto": Value Change {
        # "User modified the Auto Selection. Write to NT variable so robot knows."
        n232 = event-data() -> ("NewVal"=w364:string)  [unwired: 1 in]
        n233 = call <vilib>:"NT Write String.vi"("String"=w364, "Name"="Auto Selector") -> ()  [unwired: 9 in, 1 out]
      }
      event "Command Selection": Value Change {
        # "Get the params and show in table"
        n234 = event-data() -> ("NewVal"=w370:i32)  [unwired: 1 in]
        n235 = property on="Command Selection" class="MCListbox (strict)"() -> ("ItemNames"=w368:string[][])  [unwired: 2 in, 2 out]
        n236 = call <vilib>:"WPI_DashboardUpdate Command Params.vi"("NewVal"=w370, "Commands"=w368, "Param Tbl"=w369) -> ()  [unwired: 8 in, 1 out]
      }
      event "Execute Command": Value Change {
        # "Started one, Unique ID holds\nresponse"
        n237 = event-data() -> ()  [unwired: 1 in, 1 out]
        n238 = property on="Command Selection" class="MCListbox (strict)"() -> ("ItemNames"=w381:string[][])  [unwired: 2 in, 2 out]
        n239 = Index Array(array=w381, index (row)="Command Selection", index (col)=0) -> (element=w379:string)
        n240 = call <vilib>:"Invoke Commands.vi"("Command Params"="Command Params", "Function Name"=w379) -> ("Params"=w375:u8, "Started"=w374:bool)  [unwired: 7 in, 1 out]
        n241 = Array Subset(array="Command Params", length (row)=w375) -> (w376:string[][])  [unwired: 3 in]
        n242 = Select(t="Executing" ("Cmd Status"), s=w374, f="" ("Cmd Status")) -> (s? t:f=→"Cmd Status":string)
      }
      event "Command Selection": Double Click {
        n243 = event-data() -> ("Row"=w389:i32)  [unwired: 1 in]
        n244 = property on="Command Selection" class="MCListbox (strict)"() -> ("ItemNames"=w392:string[][])  [unwired: 2 in, 2 out]
        n245 = local read "Command Params"() -> (w388:string[][])
        n246 = Index Array(array=w392, index (row)=w389, index (col)=0) -> (element=w390:string)
        n247 = call <vilib>:"Invoke Commands.vi"("Command Params"=w388, "Function Name"=w390) -> ("Params"=w387:u8, "Started"=w382:bool)  [unwired: 7 in, 1 out]
        n248 = Array Subset(array=w388, length (row)=w387) -> (w386:string[][])  [unwired: 3 in]
        n249 = Select(t="Executing" ("Cmd Status"), s=w382, f="" ("Cmd Status")) -> (s? t:f=w383:string)
        n250 = local write "Cmd Status"(w383) -> ()
      }
      event "CheckList": Double Click {
        # "Shift clears all"
        # "Update symbols on the listbox"
        n251 = event-data() -> ("PlatMods.Shift"=w394:bool, "Row"=w396:i32)  [unwired: 1 in]
        n252 = case shown="True" w394 {
          tunnel: w396 -> [w400 _]
          tunnel: 1 -> [w399 _]
          frame False {
            n253 = property on="CheckList" class="LstBox (strict)"() -> ("Item Symbols"=w398:i32[])  [unwired: 2 in, 2 out]
            n254 = Replace Array Subset(array=w398, new element=w399, index=w400) -> (w397:i32[])
            n255 = property on="CheckList" class="LstBox (strict)"("Item Symbols"=w397) -> ()  [unwired: 2 in, 2 out]
          }
          frame True {
            w401 = 0 ("Top Row")
            n256 = property on="CheckList" class="LstBox (strict)"() -> ("Number of Rows"=w403:u32)  [unwired: 2 in, 2 out]
            n257 = Initialize Array(0, w403) -> (w402:i32[])
            n258 = property on="CheckList" class="LstBox (strict)"("Top Row"=w401, "Value"=w401, "Item Symbols"=w402) -> ()  [unwired: 2 in, 2 out]
          }
        }
      }
      event "CheckList": Key Down {
        # "Update symbols on the listbox\nLeft and right keys check and uncheck"
        n259 = event-data() -> ("VKey"=w407:T23)  [unwired: 1 in]
        n260 = case shown="\"Left\", \"Right\"" w407 {
          selector: w407 -> [w412 _]
          tunnel: eventvkey."Left" ("VKey") -> [w410 _]
          frame "Left", "Right" {
            n261 = Equal?(x=w410, y=w412) -> (x = y?=w411:bool)
            n262 = Select(t=0, s=w411, f=1) -> (s? t:f=w413:i32)
            n263 = property on="CheckList" class="LstBox (strict)"() -> ("Item Symbols"=w416:i32[])  [unwired: 2 in, 2 out]
            n264 = Replace Array Subset(array=w416, new element=w413, index="CheckList") -> (w415:i32[])
            n265 = property on="CheckList" class="LstBox (strict)"("Item Symbols"=w415) -> ()  [unwired: 2 in, 2 out]
          }
          frame Default {
          }
        }
      }
      event "Motor.Enable": Value Change {
        # "When the test mode otor enable helper is set, update that\ntree row item's value"
        n266 = event-data() -> ("NewVal"=w422:bool)  [unwired: 1 in]
        n267 = Unbundle("Motor") -> ("Value"=w421:dbl)  [unwired: 1 out]
        n268 = Select(t=w421, s=w422, f=0.0) -> (s? t:f=w419:dbl)
        n269 = call <vilib>:"NT Write Number.vi"("Numeric"=w419, "Name"=w418) -> ()  [unwired: 9 in, 1 out]
      }
      event "Test Slider": Value Change {
        # "When the test mode slider helper is set, update that\ntree row item's value"
        n270 = event-data() -> ("NewVal"=w425:dbl)  [unwired: 1 in]
        n271 = call <vilib>:"NT Write Number.vi"("Numeric"=w425, "Name"=w426) -> ()  [unwired: 9 in, 1 out]
      }
      event "On/Off": Value Change {
        # "When the test mode on/off helper value is set, update that\ntree row item's value"
        n272 = event-data() -> ("NewVal"=w430:bool)  [unwired: 1 in]
        n273 = Boolean To (0,1)(Boolean=w430) -> (0, 1=w429:i16)
        n274 = call <vilib>:"NT Write Number.vi"("Numeric"=w429, "Name"=w428) -> ()  [unwired: 9 in, 1 out]
      }
      event "Rev/Fwd": Value Change {
        # "When the test mode helper value for relays is set, update that\ntree row item's value"
        n275 = event-data() -> ("NewVal.Forward"=w438:bool, "NewVal.Reverse"=w437:bool)  [unwired: 1 in]
        n276 = Boolean To (0,1)(Boolean=w438) -> (0, 1=w434:i16)
        n277 = Boolean To (0,1)(Boolean=w437) -> (0, 1=w436:i16)
        n278 = Negate(x=w436) -> (-x=w435:i16)
        n279 = Add(x=w434, y=w435) -> (x+y=w433:i16)
        n280 = call <vilib>:"NT Write Number.vi"("Numeric"=w433, "Name"=w432) -> ()  [unwired: 9 in, 1 out]
      }
      event "Test Ring": Value Change {
        # "When a test mode helper value is selected from the ring,\nset the tree item's variable to the string value"
        n281 = event-data() -> ("NewVal"=w442:u16)  [unwired: 1 in]
        n282 = property on="Test Ring" class="Ring (strict)"() -> ("Strings []"=w443:string[])  [unwired: 2 in, 2 out]
        n283 = Index Array(array=w443, index=w442) -> (element=w441:string)
        n284 = call <vilib>:"NT Write String.vi"("String"=w441, "Name"=w440) -> ()  [unwired: 9 in, 1 out]
      }
      event "Rec Mode": Value Change {
        # "Update globals for recording mode and path to read log from.\nClear when logging and let NetworkTables set path for vision to\nuse."
        n285 = event-data() -> ("NewVal"=w454:enum32{"Stop", "Record", "Playback"})  [unwired: 1 in]
        n286 = global write "WPI_DashboardLogging Global.vi" "Logging Filename"(path "") -> ()
        n287 = global write "WPI_DashboardLogging Global.vi" "Recording"(w454) -> ()
        n288 = case shown="\"Playback\"" w454 {
          tunnel: w453 -> [_ w456 w465]
          tunnel: [_ _ w464] -> w451
          tunnel: [_ _ w463] -> _
          tunnel: w449 -> [_ _ w461]
          tunnel: cluster{i32, i32} {-250, 170} -> [_ _ w460]
          tunnel: [_ _ T24 {"Image Size"=TRUE, "Image Type"=TRUE, "Pixel Value"=TRUE, "ROI Information"=TRUE, "Zoom Factor"=FALSE} ("Image Information Shown:All Elements")] -> w444
          tunnel: [_ _ TRUE ("Zoom Factor")] -> w445
          tunnel: w447 -> [_ _ w457]
          frame Default {
          }
          frame "Stop", "Record" {
            # "Place Window too"
            n289 = invoke class="VI" method="FP.Close"(reference=w456) -> (reference out=w455:refnum<vi>)  [unwired: 2 in, 2 out]
            n290 = invoke class="VI" method="Abort VI"(reference=w455) -> ()  [unwired: 2 in, 3 out]
          }
          frame "Playback" {
            n291 = call "Open Playback Panel.vi"("Offset"=w460, "DB VI Ref"=w461, "Playback in"=w465) -> ("Playback out"=w462:refnum<vi>)  [unwired: 8 in]
            n292 = register-events(w462, w457) -> (reference out=w464:refnum<event-registration>, error out=w463:errorcluster)  [unwired: 2 in]
          }
        }
        n293 = property on="Camera Image Right" class="ImageControl"("Image Information Shown"=w444, "Image Information Visible"=w445) -> ()  [unwired: 2 in, 2 out]
        n294 = property on="Camera Image" class="ImageControl"("Image Information Shown"=w444, "Image Information Visible"=w445) -> ()  [unwired: 2 in, 2 out]
        n295 = call <vilib>:"WPI_DashboardNT Log FieldName Cache.vi"("Operation"=enum16{"Lookup/Add", "Index", "Clear"}."Clear") -> ()  [unwired: 8 in, 3 out]
      }
      event Panel Close {
        w467 = enum32{"Stop", "Record", "Playback"}."Stop" ("Rec Mode")
        # "Playback window has been closed, abort"
        n296 = event-data() -> ()  [unwired: 1 in, 4 out]
        n297 = local write "Rec Mode"(w467) -> ()
        n298 = global write "WPI_DashboardLogging Global.vi" "Recording"(w467) -> ()
      }
      event Panel Close {
        # "Abort playback window and ourself"
        n299 = event-data() -> ()  [unwired: 1 in, 4 out]
        n300 = invoke class="VI" method="FP.Close"(reference=w471) -> (reference out=w470:refnum<vi>)  [unwired: 2 in, 2 out]
        n301 = invoke class="VI" method="Abort VI"(reference=w470) -> (error out=w469:errorcluster)  [unwired: 2 in, 2 out]
        n302 = invoke class="VI" method="Abort VI"(error in=w469) -> ()  [unwired: 2 in, 3 out]
      }
      event User Event {
        n303 = event-data() -> ("IDs"=w478:cluster{"RPC field ID":u16, "Unique ID":u16}, "String"=w477:string)  [unwired: 1 in]
        n304 = Bundle("IDs"=w478, "String"=w477) -> (w476:T10)  [unwired: 1 in]
        n305 = call <vilib>:"Retrieve RPC Response.vi"("RPC Response"=w476) -> ("Output"=w474:string[][])  [unwired: 10 in]
        n306 = Build Array (concatenate)(w472, w474) -> (w473:string[][])
        n307 = local write "Command Params"(w473) -> ()
        n308 = local write "Cmd Status"("" ("Cmd Status")) -> ()
      }
      event "Tree": Double Click {
        n309 = event-data() -> ("PlatMods"=w484:T27, "Tag"=w481:string)  [unwired: 1 in]
        n310 = Unbundle(w484) -> ("Shift"=w483:bool)  [unwired: 4 out]
        n311 = String Subset(string=w481, length (rest)=1 ("length (rest)")) -> (substring=w480:string)  [unwired: 1 in]
        n312 = Not(x=w483) -> (.not. x?=w482:bool)
        n313 = case shown="\"/\"" w480 {
          tunnel: w481 -> [_ w487]
          tunnel: w482 -> [_ w486]
          frame Default {
          }
          frame "/" {
            n314 = call <vilib>:"NT Update Persistence.vi"("Persistence"=w486, "Name"=w487) -> ()  [unwired: 9 in, 1 out]
          }
        }
      }
    }
  }
  n315 = while {
    tunnel: w65 -> [w489]
    i -> [w492]
    stop <- FALSE stop-if-true
    n316 = Wait (ms)(milliseconds to wait=u32 100) -> ()  [unwired: 1 out]
    n317 = case shown="\"Playback\"" "Rec Mode" {
      tunnel: w492 -> [_ _ w507]
      tunnel: [u32 2829099 ("Base Color") u32 11141120 ("Target Color") w496] -> w488
      frame "Stop", Default {
        # "Reset the color, extra updates don't cost much"
      }
      frame "Record" {
      }
      frame "Playback" {
        # "Playback"
        n318 = Quotient & Remainder(x=w507, y=u32 50 ("milliseconds to wait")) -> (x-y*floor(x/y)=w503:u32)  [unwired: 1 out]
        n319 = Divide(x=w503, y=u32 50 ("milliseconds to wait")) -> (x/y=w500:dbl)
        n320 = Multiply(x=6.283185307179586, y=w500) -> (x*y=w505:dbl)
        n321 = Sine(x=w505) -> (sin(x)=w504:dbl)
        n322 = Absolute Value(x=w504) -> (abs(x)=w497:dbl)
        n323 = call "Interpolate RGB Color.vi"("Proportion"=w497, "Target Color"=u32 30976, "Base Color"=u32 2829099) -> ("Result Color"=w496:u32)  [unwired: 8 in]
      }
    }
    n324 = property class="Pane"(reference=w489, "PaneColor"=w488) -> ()  [unwired: 1 in, 2 out]
  }
  n325 = local write "Dashboard Tab"(T8."Drive" ("Dashboard Tab")) -> ()
  n326 = property on="On/Off" class="Bool (strict)"("Visible"=w36) -> ()  [unwired: 2 in, 2 out]
  n327 = property on="Motor" class="Clust (strict)"("Visible"=w36) -> ()  [unwired: 2 in, 2 out]
  n328 = property on="Progress" class="Clust (strict)"("Visible"=w36) -> ()  [unwired: 2 in, 2 out]
  n329 = property on="Test Ring" class="Ring (strict)"("Visible"=w36) -> ()  [unwired: 2 in, 2 out]
  n330 = property on="Rev/Fwd" class="Clust (strict)"("Visible"=w36) -> ()  [unwired: 2 in, 2 out]
  n331 = while {
    tunnel: u16 1741 ("timeout ms (25000)") -> [w509]
    stop <- FALSE stop-if-true
    n332 = TCP Create Listener(10:w509) -> (0:w508:errorcluster, 3:w510:refnum<k5>)  [unwired: 4 in, 1 out]
    n333 = case shown="No Error" w508 {
      selector: w508 -> [w512 _]
      tunnel: w510 -> [w513 _]
      frame No Error {
        n334 = while {
          tunnel: w513 -> [w516]
          tunnel: w512 -> [w515]
          stop <- FALSE stop-if-true
          n335 = TCP Wait On Listener(8:w515, 11:w516) -> (0:w517:errorcluster, 4:w518:refnum<k5>)  [unwired: 2 in, 3 out]
          n336 = local write "TCP"(w518) -> ()
          n337 = case shown="No Error" w517 {
            frame No Error {
            }
            frame Error {
              n338 = Wait (ms)(milliseconds to wait=u32 1000) -> ()  [unwired: 1 out]
            }
          }
        }
      }
      frame Error {
        n339 = Wait (ms)(milliseconds to wait=u32 1000) -> ()  [unwired: 1 out]
      }
    }
  }
  n340 = local write "Command Selection"(u16 0 ("milliseconds to wait")) -> ()
  n341 = local write "Command Params"(string[][] [] ("Command Params")) -> ()
  n342 = global write "WPI_DashboardLogging Global.vi" "Recording"(w59) -> ()
  n343 = local write "Rec Mode"(w59) -> ()
  n344 = call <vilib>:"NT Write String.vi"("String"="Select Auto", "Name"="Auto Selector") -> ()  [unwired: 9 in, 1 out]
